vi "Do.vi"(8 "error in (no error)":errorcluster, 10 "Actor in":refnum<class "Actor.lvclass">, 11 "Clear History Msg":refnum<class "Clear History Msg.lvclass">) -> (0 "error out":errorcluster, 2 "Actor out":refnum<class "Actor.lvclass">)   [LabVIEW 2019, in "BNT_XtGraph.lvlib" / "Clear History Msg.lvclass"]
doc: "This VI delivers the message to the actor by calling the appropriate method(s) on the actor."
uses:
  Clear History Msg.lvclass
  BNT_XtGraph/BNT_XtGraph.lvclass
  CSPP_Core/Messages/CSPP_AsyncCallbackMsg/CSPP_AsyncCallback Msg.lvclass
  C:/Program Files (x86)/National Instruments/LabVIEW 2018/vi.lib/ActorFramework/Actor/Actor.lvclass
  <vilib>/ActorFramework/Actor/Actor.lvclass
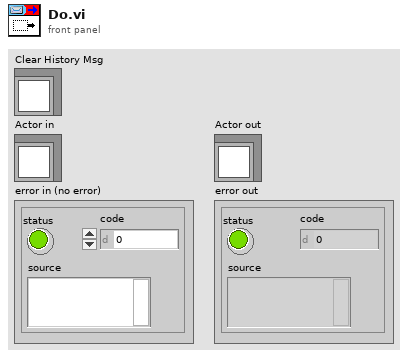
[diagram p1: front panel]
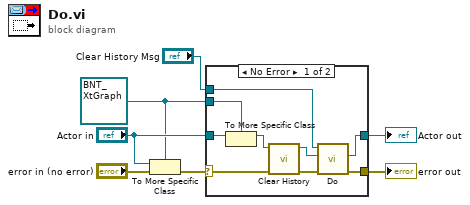
[diagram p0: block diagram]
diagram:
  w2 = refnum<class "BNT_XtGraph.lvclass"> refnum ("Actor in")
  n1 = To More Specific Class(target class=w2, reference="Actor in", error in="error in (no error)") -> (error out=w6:errorcluster)  [unwired: 1 out]
  n2 = case shown="No Error" w6 {
    selector: w6 -> [w16 w18]
    tunnel: [w12 w18] -> w5
    tunnel: [w11 w17] -> w4
    tunnel: "Actor in" -> [w15 w17]
    tunnel: w2 -> [w14 _]
    tunnel: "Clear History Msg" -> [w8 _]
    frame No Error {
      n3 = To More Specific Class ("To More Specific Class (internal)")(target class=w14, reference=w15) -> (specific class reference=w13:refnum<class "BNT_XtGraph.lvclass">)  [unwired: 1 in, 1 out]
      n4 = call "Clear History.vi"("Error In"=w16, "BNT_XtGraph in"=w13) -> ("Error Out"=w9:errorcluster, "BNT_XtGraph out"=w10:refnum<class "BNT_XtGraph.lvclass">)  [unwired: 8 in]
      n5 = call-parent "Do.vi"("error in (no error)"=w9, "Actor in"=w10, "CSPP_AsyncCallback Msg"=w8) -> ("error out"=w12:errorcluster, "Actor out"=w11:refnum<class "Actor.lvclass">)  [unwired: 7 in]
    }
    frame Error {
    }
  }
  "error out" <- w5
  "Actor out" <- w4
